vi "PR_Check_All .vi"(8 "error in (no error)":errorcluster, 9 "測高使不使用":bool, 10 "barcode":string="981321652", 11 "DBlink":string="Driver={ODBC Driver 17 for SQL Server};Server=localhost\\SQLEXPRESS;Database=ZDX201;UID=labview;PWD=Dsa@54137926") -> (0 "error out":errorcluster, 2 "結果":string="OK", 3 "ToPLC":u32)   [LabVIEW 2019]
uses:
  <vilib>/addons/database/Connection.llb/DB Tools Open Connec (String).vi
  <vilib>/addons/database/Connection.llb/Conn Execute.vi
  <vilib>/addons/database/Recordset.llb/Rec Fetch Recordset Data (R).vi
  <vilib>/addons/database/Recordset.llb/Rec Destroy - Connection.vi
  <vilib>/addons/database/_DB Variant To Data/Database Variant To Data.xnode
  <vilib>/addons/database/NI_Database_API.lvlib
panel:
  out "Final Result":bool[](array[boolean])
  out "ESR":bool
  out "SR":bool
  out "eve_screw_result":string
  out "screw_result":string
  out "data":T1(array[cluster])
  out "查詢結果":string="SELECT \n       [barcode A]\n      ,[barcode B]\n  FROM [ZDX201].[dbo].[workplace_data]\n  where [workplace_name_id]>9 and [workplace_name_id]<11 and ([barcode A] is not null or [barcode B] is not null)\n  order by [workplace_name_id]"
  # "0: 兩者皆NG\n1: 僅扭力過關\n2: 僅螺絲檢測過關\n3: OK"
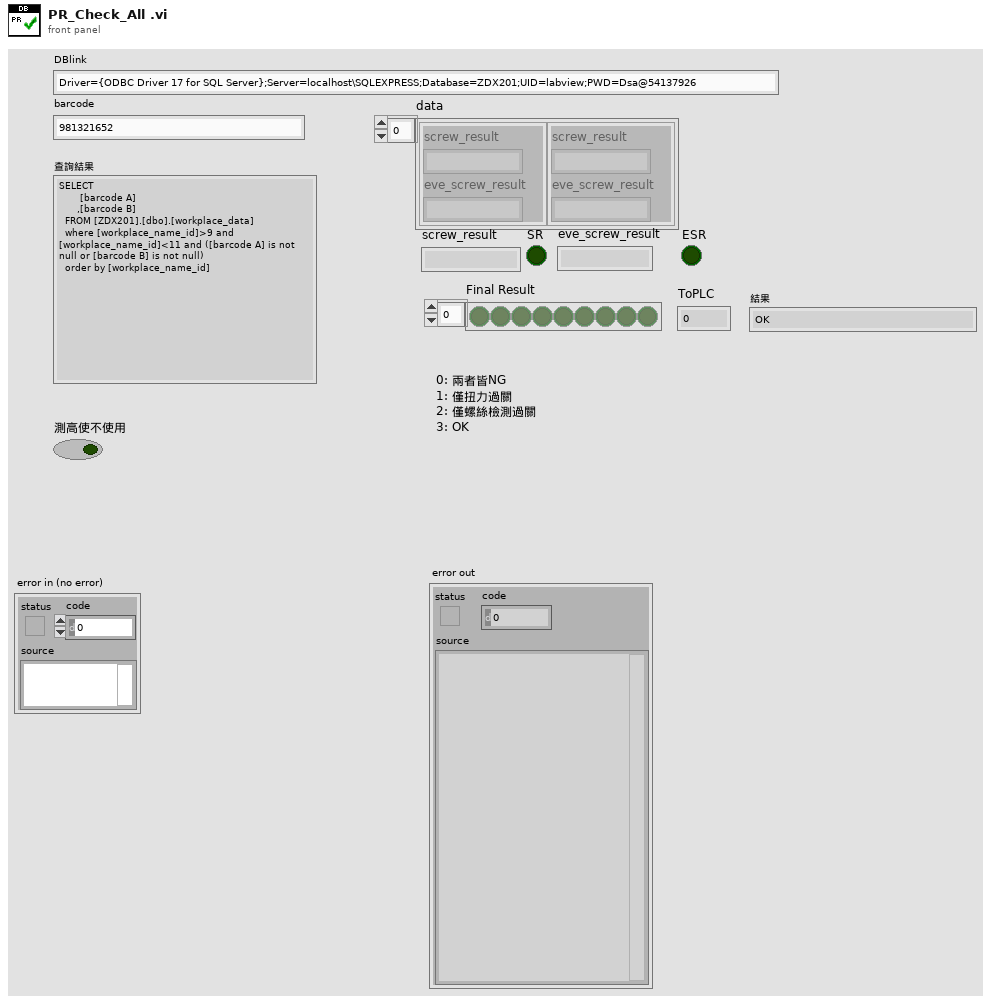
[diagram p1: front panel]
types:
  T1 = cluster{"screw_result":string, "eve_screw_result":string}[]
  T2 = cluster{"[time_spout]":timestamp, "update_time":timestamp, "[workspace_id]":i32, "QC_result":string}
  T3 = typedef "NI_Database_API.lvlib/Conn ObjectReference.ctl" = refnum<k1>
  T4 = typedef "NI_Database_API.lvlib/Rec ObjectReference.ctl" = refnum<k1>
  T5 = cluster{"screw_result":string, "eve_screw_result":string}
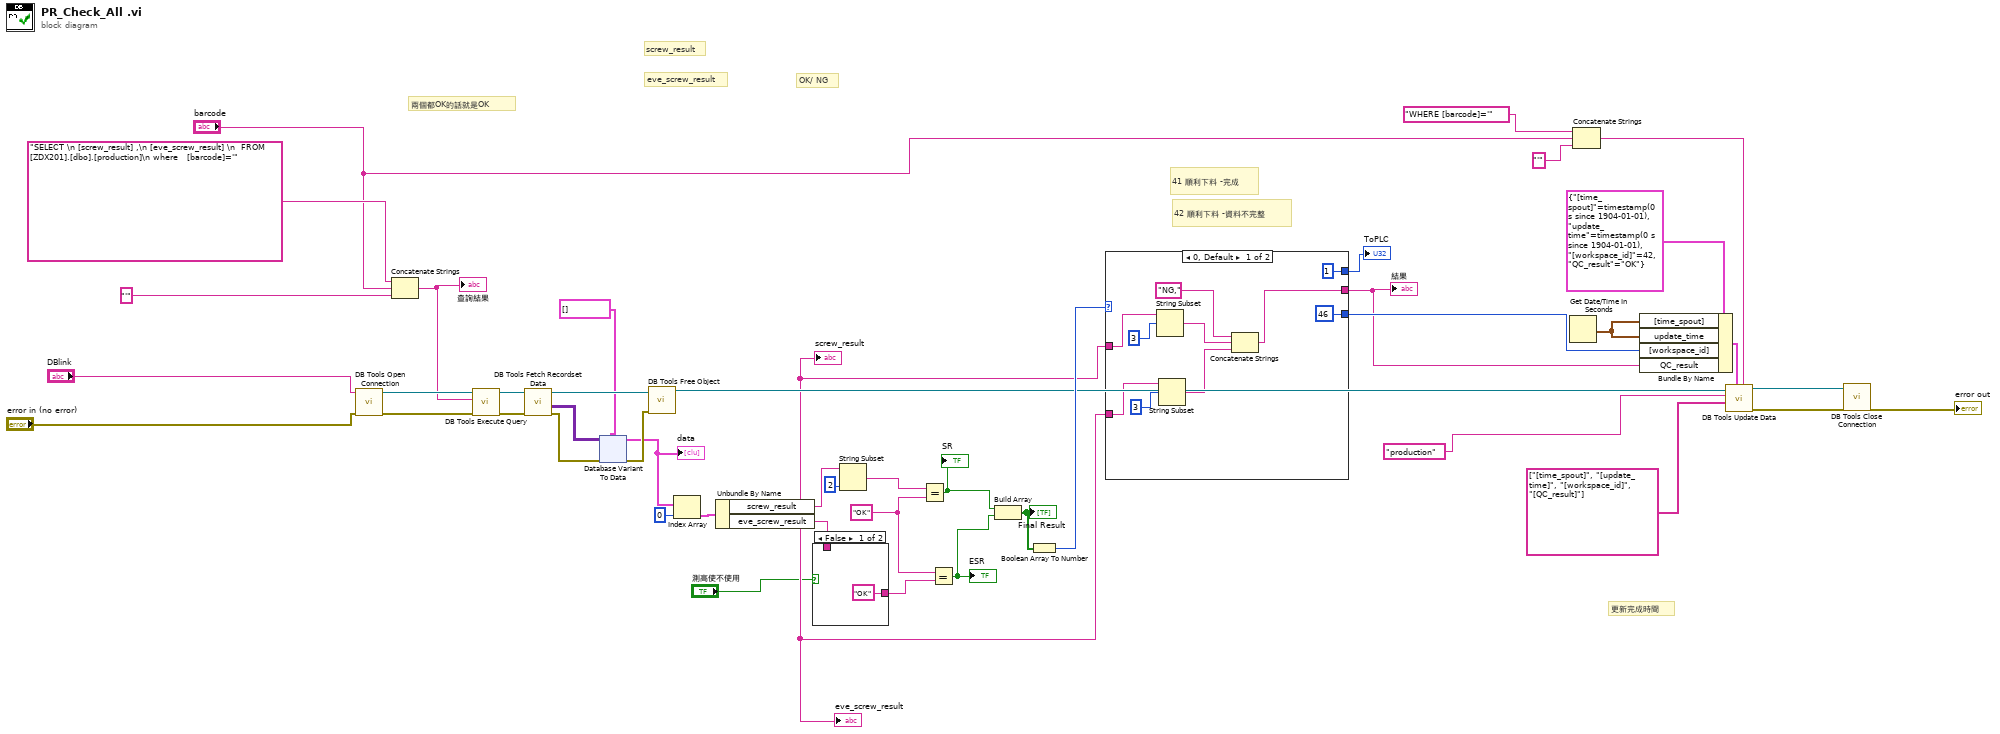
[diagram p0: block diagram]
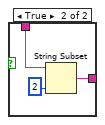
[diagram p2: hidden frame]
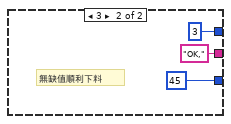
[diagram p3: hidden frame]
diagram:
  w24 = "OK" ("x")
  # "42\t順利下料 -資料不完整"
  # "41\t順利下料 -完成"
  # "更新完成時間"
  # "OK/ NG"
  # "兩個都OK的話就是OK"
  # "eve_screw_result"
  # "screw_result"
  n1 = call-poly <vilib>:"DB Tools Open Connection.vi"("error in (no error)"="error in (no error)", "connection information"="DBlink") -> ("error out"=w42:errorcluster, "connection reference"=w41:T3)  [unwired: 6 in]
  n2 = Concatenate Strings("SELECT \n [screw_result] ,\n [eve_screw_result] \n  FROM [ZDX201].[dbo].[production]\n where   [barcode]='", "barcode", "'" ("string")) -> (w33:string)
  "查詢結果" <- w33
  n3 = call-poly <vilib>:"DB Tools Execute Query.vi"("error in (no error)"=w42, "SQL query"=w33, "connection reference"=w41) -> ("error out"=w39:errorcluster, "recordset reference"=w40:T4)  [unwired: 5 in]
  n4 = call-poly <vilib>:"DB Tools Fetch Recordset Data.vi"("error in (no error)"=w39, "recordset reference"=w40) -> ("error out"=w36:errorcluster, "recordset data"=w35:variant[][], "recordset reference out"=w37:T4)  [unwired: 3 in]
  n5 = xnode "Database Variant To Data"("database variant"=w35, "error in (no error)"=w36, "type"=T1 [] ("subarray")) -> ("data"=w27:T1, "error out"=w38:errorcluster)
  "data" <- w27
  n6 = call-poly <vilib>:"DB Tools Free Object.vi"("error in (no error)"=w38, "recordset reference"=w37) -> ("connection reference"=w8:T3)  [unwired: 8 in, 1 out]
  n7 = Index Array(array=w27, index=0) -> (element=w25:T5)
  n8 = Unbundle By Name(w25) -> ("screw_result"=w5:string, "eve_screw_result"=w4:string)
  "screw_result" <- w5
  "eve_screw_result" <- w4
  n9 = case shown="False" "測高使不使用" {
    tunnel: w4 -> [_ w47]
    tunnel: ["OK" ("eve_screw_result") w46] -> w3
    frame False {
    }
    frame True {
      n10 = String Subset(string=w47, length (rest)=2 ("length (rest)")) -> (substring=w46:string)  [unwired: 1 in]
    }
  }
  n11 = String Subset(string=w5, length (rest)=2 ("length (rest)")) -> (substring=w6:string)  [unwired: 1 in]
  n12 = Equal?(x=w6, y=w24) -> (x = y?=w23:bool)
  "SR" <- w23
  n13 = Equal?(x=w24, y=w3) -> (x = y?=w22:bool)
  "ESR" <- w22
  n14 = Build Array(w23, w22) -> (w21:bool[])
  "Final Result" <- w21
  n15 = Boolean Array To Number(Boolean array=w21) -> (number=w9:u32)
  n16 = case shown="0, Default" w9 {
    tunnel: [46 45] -> w12
    tunnel: [w49 "OK," ("組合結果")] -> w10
    tunnel: w5 -> [w55 _]
    tunnel: w4 -> [w53 _]
    tunnel: [u32 1 ("ToPLC") u32 3 ("ToPLC")] -> w2
    frame 0, Default {
      n17 = String Subset(string=w55, offset (0)=3 ("length (rest)")) -> (substring=w52:string)  [unwired: 1 in]
      n18 = String Subset(string=w53, offset (0)=3 ("length (rest)")) -> (substring=w51:string)  [unwired: 1 in]
      n19 = Concatenate Strings("NG," ("組合結果"), w52, w51) -> (w49:string)
    }
    frame 3 {
      # "無缺值順利下料"
    }
  }
  "ToPLC" <- w2
  "結果" <- w10
  n20 = Get Date/Time In Seconds() -> (seconds since 1Jan1904=w18:timestamp)
  n21 = Concatenate Strings("WHERE [barcode]='", "barcode", "'" ("string")) -> (w14:string)
  n22 = Bundle By Name(cluster=T2 {"[time_spout]"=timestamp(0 s since 1904-01-01), "update_time"=timestamp(0 s since 1904-01-01), "[workspace_id]"=42, "QC_result"="OK"} ("input cluster"), "[time_spout]"=w18, "update_time"=w18, "[workspace_id]"=w12, "QC_result"=w10) -> (w20:T2)
  n23 = call <vilib>:"DB Tools Update Data.vi"("condition"=w14, "data"=w20, "columns"=string[] ["[time_spout]", "[update_time]", "[workspace_id]", "[QC_result]"], "table"="production", "connection reference"=w8) -> ("error out"=→"error out":errorcluster, "connection reference out"=w13:T3)  [unwired: 5 in]
  n24 = call <vilib>:"DB Tools Close Connection.vi"("connection reference"=w13) -> ()  [unwired: 6 in, 1 out]
